vi "mod_Continuous BB-CPM generation.vi"(0 "Bit stream":T2(tab), 1 "Symbol Rate, Hz":dbl=1.0 format="%.2f", 2 "CPM system parameters":T3={"samples per symbol (16)"=1, "symbol map"=[]}, 5 "PN Sequence Order":i32=9, 7 "filter type":T1(ring), 9 "user base bit pattern":i8[](array[numeric]), 11 "error in (no error)":errorcluster, 12 "Filter Length":i32=6, 13 "Path":path, 14 "filter parameter":dbl=0.5 format="%.2f") -> (4 "data complex waveform":T4 {"Y" format="%.3f"; "dt" format="%^.2e"; "t0" format="%.4f"}, 15 "error out":errorcluster)   [LabVIEW 2020, in "niDMT.lvlib"]
uses:
  <vilib>/addons/Modulation/niDMT.lvlib
  <vilib>/addons/Modulation/Analog/controls/Complex Data Waveform.ctl
  <vilib>/addons/Modulation/Digital/Support/Controls/CPM System Parameters.ctl
  <vilib>/addons/Modulation/Digital/General/MT Generate Bits (Galois, PN Order).vi
  <vilib>/addons/Modulation/Digital/Support/Common/Validators/mod_Generate Bits Validate.vi
  <vilib>/addons/Modulation/Analog/support/mod_Set Error Source.vi
  <vilib>/addons/Modulation/Digital/General/subVIs/mod_Generate Bits PN Sequence.vi
  <vilib>/addons/Modulation/Digital/General/MT Generate Bits (User Defined).vi
  <vilib>/Utility/file.llb/Read From Spreadsheet File (DBL).vi
  <vilib>/addons/Modulation/Digital/Support/Common/Validators/mod_Generate Filter Coefficients Validate.vi
  <vilib>/addons/Modulation/Digital/General/subVIs/mod_Generate Filter Coefficients.vi
  <vilib>/addons/Modulation/niAMT.lvlib
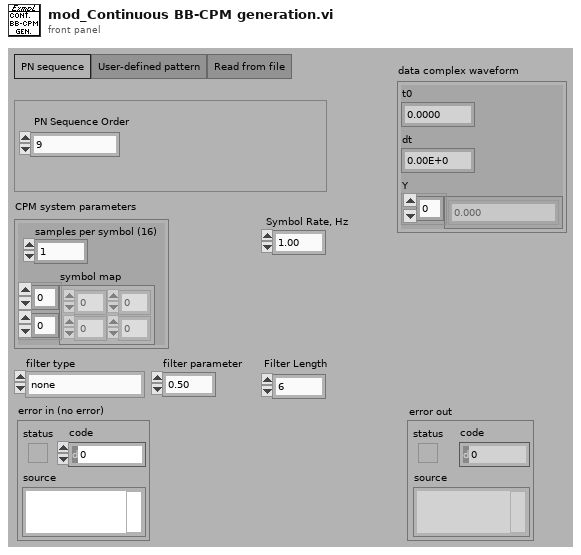
[diagram p1: front panel]
types:
  T1 = enum16{"none", "Raised Cosine", "Root Raised Cos", "Gaussian"}
  T2 = enum32{"PN sequence", "User-defined pattern", "Read from file"}
  T3 = typedef "niDMT.lvlib/CPM System Parameters.ctl" = cluster{"samples per symbol (16)":i32, "symbol map":dbl[][]}
  T4 = typedef "niAMT.lvlib/Complex Data Waveform.ctl" = cluster{"t0":dbl, "dt":dbl, "Y":cdb[]}
  T5 = enum16{"FSK", "PSK", "QAM", "MSK", "PAM", "ASK", "CPM"}
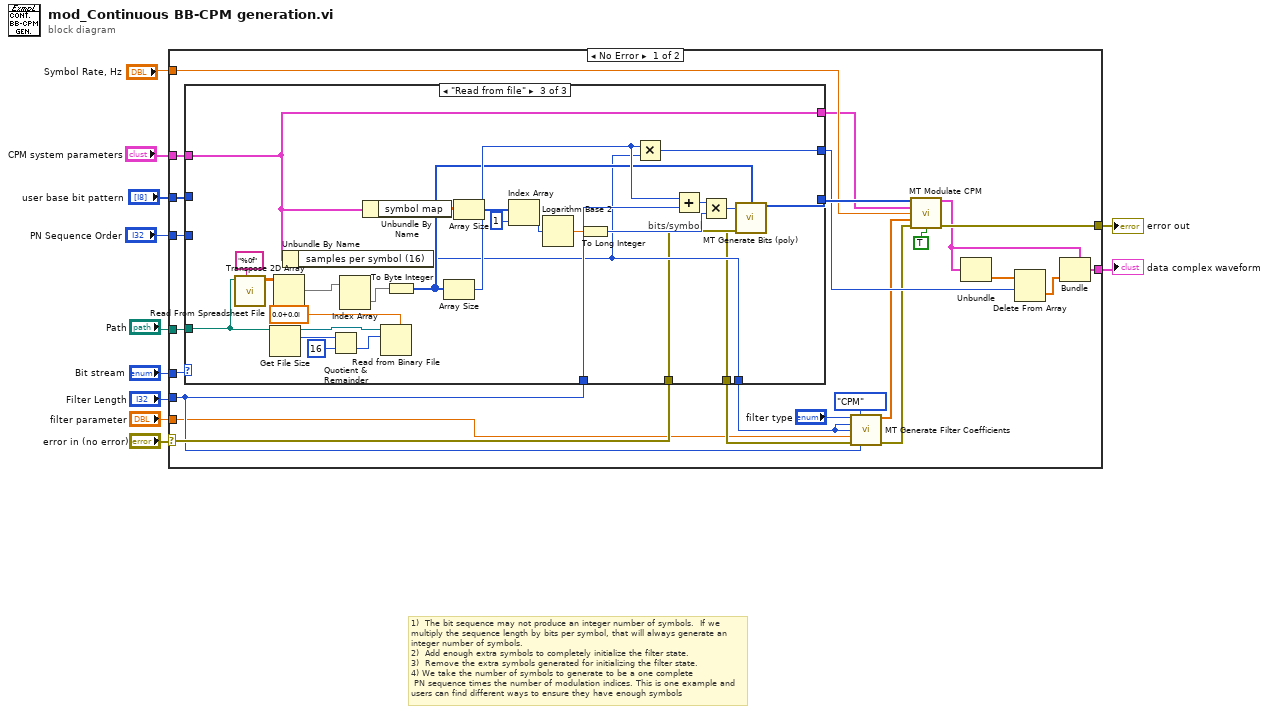
[diagram p0: block diagram]
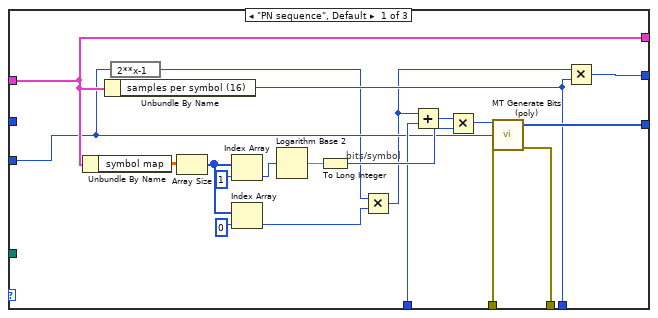
[diagram p2: hidden frame]
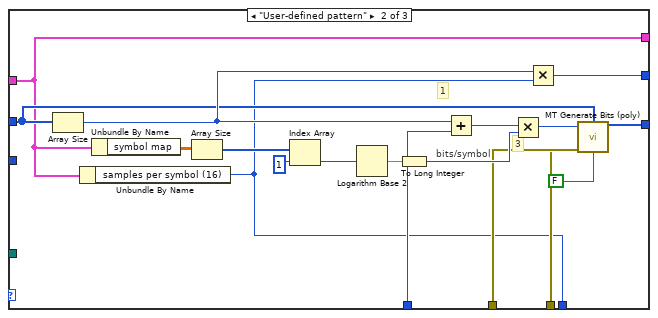
[diagram p3: hidden frame]
diagram:
  # "1)  The bit sequence may not produce an integer number of symbols.  If we multiply the sequence length by bits per symbol, that will always generate an integer number of symbols. \n2)  Add enough extra symbols to completely initialize the filter state.\n3)  Remove the extra symbols generated for initializing the filter state. \n4) We take the number of symbols to generate to be a one complete\n PN sequence times the number of modulation indices. This is one example and users can find different ways to ensure they have enough symbols"
  n1 = case shown="No Error" "error in (no error)" {
    selector: "error in (no error)" -> [w28 w101]
    tunnel: [w35 _] -> w11
    tunnel: [w27 w101] -> w10
    tunnel: "Symbol Rate, Hz" -> [w15 _]
    tunnel: "PN Sequence Order" -> [w30 _]
    tunnel: "user base bit pattern" -> [w34 _]
    tunnel: "Bit stream" -> [w32 _]
    tunnel: "Filter Length" -> [w20 _]
    tunnel: "CPM system parameters" -> [w29 _]
    tunnel: "Path" -> [w31 _]
    tunnel: "filter parameter" -> [w17 _]
    frame No Error {
      n2 = case shown="\"Read from file\"" w32 {
        tunnel: w34 -> [_ w65 _]
        tunnel: w30 -> [w41 _ _]
        tunnel: w31 -> [_ _ w81]
        tunnel: w29 -> [w52 w63 w87]
        tunnel: [w44 w57 w89] -> w22
        tunnel: [w47 w68 w88] -> w16
        tunnel: w20 -> [w42 w66 w90]
        tunnel: [w45 w64 w76] -> w26
        tunnel: [w52 w63 w87] -> w14
        tunnel: w28 -> [w51 w62 w86]
        tunnel: [w50 w61 w85] -> w21
        frame "PN sequence", Default {
          # "bits/symbol"
          n3 = Unbundle By Name(w52) -> ("symbol map"=w53:dbl[][])
          n4 = Unbundle By Name(w52) -> ("samples per symbol (16)"=w44:i32)
          n5 = expression code="2**x-1"(w41) -> (w37:i32)
          n6 = Array Size(array=w53) -> (size(s)=w39:i32[])
          n7 = Index Array(array=w39, index=1) -> (element=w49:i32)
          n8 = Index Array(array=w39, index=0) -> (element=w38:i32)
          n9 = Logarithm Base 2(1:w49) -> (0:w54:dbl)
          n10 = To Long Integer(number=w54) -> (32bit integer=w46:i32)
          n11 = Multiply(x=w37, y=w38) -> (x*y=w36:i32)
          n12 = Add(x=w36, y=w42) -> (x+y=w43:i32)
          n13 = Multiply(x=w43, y=w46) -> (x*y=w55:i32)
          n14 = call-poly <vilib>:"MT Generate Bits (poly).vi"("total bits (128)"=w55, "PN sequence order (9)"=w41, "error in (no error)"=w51) -> ("output bit stream"=w45:i8[], "error out"=w50:errorcluster)  [unwired: 2 in, 9 out]
          n15 = Multiply(x=w36, y=w44) -> (x*y=w47:i32)
        }
        frame "User-defined pattern" {
          # "1"
          # "3"
          # "bits/symbol"
          n16 = Array Size(array=w65) -> (size(s)=w67:i32)
          n17 = Unbundle By Name(w63) -> ("samples per symbol (16)"=w57:i32)
          n18 = Unbundle By Name(w63) -> ("symbol map"=w69:dbl[][])
          n19 = Array Size(array=w69) -> (size(s)=w59:i32[])
          n20 = Index Array(array=w59, index=1) -> (element=w58:i32)
          n21 = Logarithm Base 2(1:w58) -> (0:w70:dbl)
          n22 = To Long Integer(number=w70) -> (32bit integer=w71:i32)
          n23 = Add(x=w67, y=w66) -> (x+y=w72:i32)
          n24 = Multiply(x=w72, y=w71) -> (x*y=w73:i32)
          n25 = Multiply(x=w67, y=w57) -> (x*y=w68:i32)
          n26 = call-poly <vilib>:"MT Generate Bits (poly).vi"("total bits (128)"=w73, "user base bit pattern"=w65, "error in (no error)"=w62, "reset? (T)"=FALSE) -> ("output bit stream"=w64:i8[], "error out"=w61:errorcluster)  [unwired: 1 in, 9 out]
        }
        frame "Read from file" {
          # "bits/symbol"
          n27 = call-poly <vilib>:"Read From Spreadsheet File.vi"("format (%.3f)"="%0f", "file path (dialog if empty)"=w81) -> ("all rows"=w99:dbl[][])  [unwired: 2 in, 7 out]
          n28 = Get File Size(file=w81) -> (refnum out=w80:refnum<file>, size (in bytes)=w79:i64)  [unwired: 1 in, 1 out]
          n29 = Transpose 2D Array(2D array=w99) -> (transposed array=w74:dbl[][])
          n30 = Unbundle By Name(w87) -> ("samples per symbol (16)"=w89:i32)
          n31 = Quotient & Remainder(x=w79, y=i64 16) -> (floor(x/y)=w77:i64)  [unwired: 1 out]
          n32 = Index Array(array=w74) -> (element=w100:dbl[])  [unwired: 2 in]
          n33 = Unbundle By Name(w87) -> ("symbol map"=w93:dbl[][])
          n34 = Read from Binary File(5:cdb 0.0+0.0i, 10:w77, 11:w80) -> ()  [unwired: 2 in, 5 out]
          n35 = To Byte Integer(number=w100) -> (8bit integer=w91:i8[])
          n36 = Array Size(array=w91) -> (size(s)=w92:i32)
          n37 = Array Size(array=w93) -> (size(s)=w75:i32[])
          n38 = Index Array(array=w75, index=1) -> (element=w83:i32)
          n39 = Logarithm Base 2(1:w83) -> (0:w94:dbl)
          n40 = To Long Integer(number=w94) -> (32bit integer=w95:i32)
          n41 = Multiply(x=w92, y=w89) -> (x*y=w88:i32)
          n42 = Add(x=w92, y=w90) -> (x+y=w96:i32)
          n43 = Multiply(x=w96, y=w95) -> (x*y=w97:i32)
          n44 = call-poly <vilib>:"MT Generate Bits (poly).vi"("total bits (128)"=w97, "user base bit pattern"=w91, "error in (no error)"=w86) -> ("output bit stream"=w76:i8[], "error out"=w85:errorcluster)  [unwired: 2 in, 9 out]
        }
      }
      n45 = call <vilib>:"MT Generate Filter Coefficients.vi"("pulse shaping filter (none)"="filter type", "modulation type"=T5."CPM", "pulse shaping samples per symbol (16)"=w22, "matched samples per symbol (16)"=w22, "filter parameter"=w17, "error in (no error)"=w21, "filter length (symbols)"=w20) -> ("pulse shaping filter coefficients"=w13:dbl[], "error out"=w12:errorcluster)  [unwired: 7 out]
      n46 = call <vilib>:"MT Modulate CPM.vi"("input bit stream"=w26, "CPM system parameters"=w14, "symbol rate (Hz)"=w15, "pulse shaping filter coefficients"=w13, "error in (no error)"=w12, "reset? (T)"=TRUE ("Reset (T)")) -> ("output complex waveform"=w24:T4, "error out"=w27:errorcluster)  [unwired: 1 in, 7 out]
      n47 = Unbundle(w24) -> ("Y"=w33:cdb[])  [unwired: 2 out]
      n48 = Delete From Array(array=w33, length=w16) -> (deleted portion=w23:cdb[])  [unwired: 1 in, 1 out]
      n49 = Bundle(cluster=w24, "Y"=w23) -> (w35:T4)  [unwired: 2 out]
    }
    frame Error {
    }
  }
  "error out" <- w10
  "data complex waveform" <- w11
